vi "TSCAN_TestDBC.vi"() -> (3 "SigValue":i32)   [LabVIEW 2019]
panel:
  out "x = 0?":bool
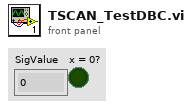
[diagram p1: front panel]
types:
  T1 = cluster{"Data0":u8, "Data1":u8, "Data2":u8, "Data3":u8, "Data4":u8, "Data5":u8, "Data6":u8, "Data7":u8}
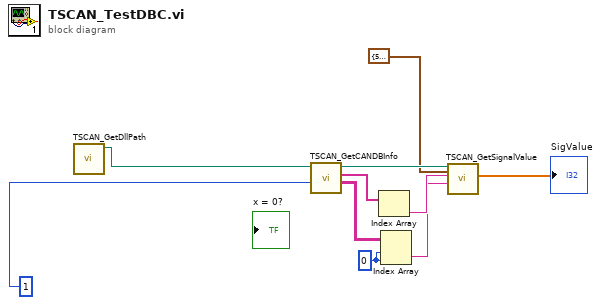
[diagram p0: block diagram]
diagram:
  w5 = 0 ("禁用的索引 (列)")
  n1 = call "TSCAN_GetDllPath.vi"() -> ("DllPath"=w10:path)  [unwired: 11 in]
  n2 = call "TSCAN_GetCANDBInfo.vi"("ADatabaseld"=u32 1 ("AIdIn"), "路径输入"=w10) -> ("SignalName"=w6:string[][], "Message"=w7:string[], "路径输出"=w8:path)  [unwired: 7 in]
  n3 = Index Array(array=w7) -> (element=w2:string)  [unwired: 1 in]
  n4 = Index Array(array=w6, index (row)=w5, index (col)=w5) -> (element=w1:string)
  n5 = call "TSCAN_GetSignalValue.vi"("ALLID"=T1 {"Data0"=55, "Data1"=124, "Data2"=39, "Data3"=16, "Data4"=0, "Data5"=0, "Data6"=0, "Data7"=0} ("ADataArray"), 9:w1, 10:w2, "路径输入"=w8) -> ("SigValue"=→"SigValue":dbl[])  [unwired: 4 in, 3 out]
